vi "IncrementalMove.vi"() -> ()   [LabVIEW 2019]
uses:
  <vilib>/userDefined/High Color/IMAQdx.ctl
  <vilib>/vision/driver/NI_Vision_Acquisition_Software.lvlib
  <vilib>/vision/NI_Vision_Development_Module.lvlib
panel:
  in  "ShowCam":bool
  in  "milliseconds to wait":u32=500
  in  "BadImage":bool
  out "Position_XYZ":string
  out "Gcode":string
  in  "Relative":bool=TRUE
  in  "Z":dbl
  in  "Y":dbl
  in  "X":dbl
  in  "Axis":enum16{"X", "Y", "Z"}(ring)
  out "Image":T1(plugin-control)
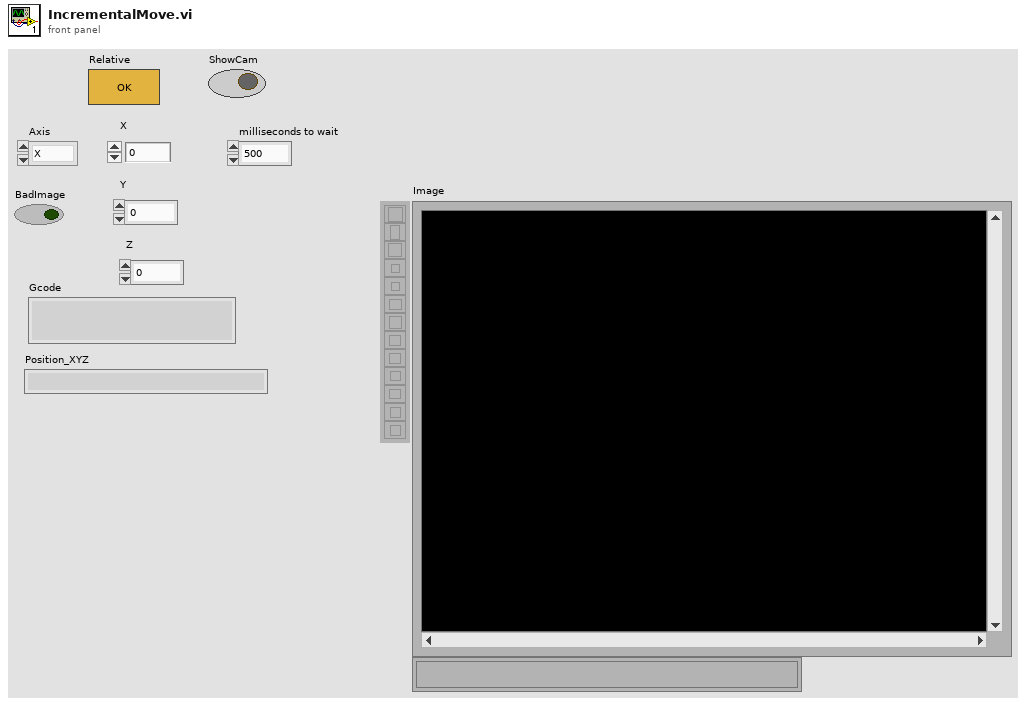
[diagram p1: front panel]
types:
  T1 = typedef "IMAQ Image.ctl" = refnum<image>
  T2 = typedef "IMAQ Circle" = cluster{"Center X":i32, "Center Y":i32, "Inner Radius":i32, "Outer Radius":i32, "Start Angle":dbl, "End Angle":dbl}
  T3 = typedef "IMAQdx.ctl" = refnum<k21>
  T4 = typedef "Image Type" = u32
  T5 = typedef "ROI Descriptor" = cluster{"Global Rectangle":i32[], "Contours":cluster{"ID":enum32{"External", "Internal"}, "Type":u32, "Coordinates":i32[]}[]}
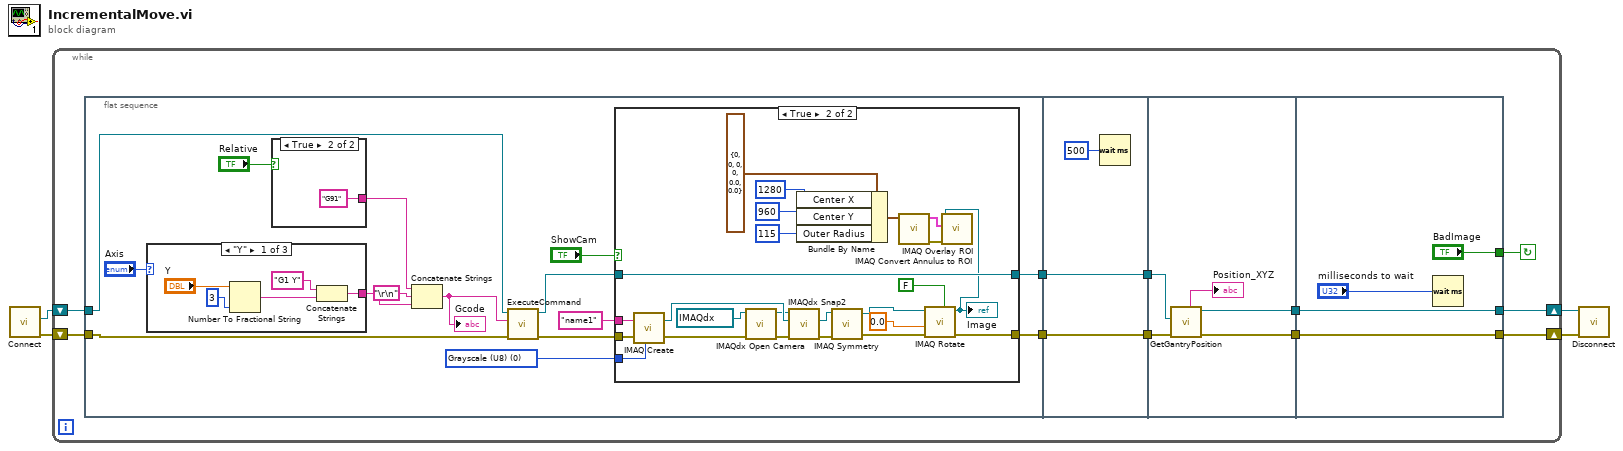
[diagram p0: block diagram]
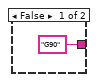
[diagram p3: hidden frame]
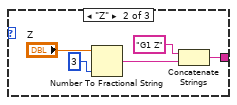
[diagram p4: hidden frame]
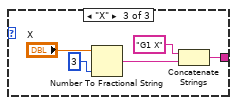
[diagram p5: hidden frame]
diagram:
  n1 = call "Connect.vi"() -> ("error out"=w4:errorcluster, "controller"=w3:refnum<k24>)  [unwired: 10 in]
  n2 = while {
    shift-right: [w13] -> w2
    shift-left: w4 -> [w15]
    shift-right: [w12] -> w1
    shift-left: w3 -> [w14]
    stop <- w11 continue-if-true
    n3 = flat-sequence {
      tunnel: w15 -> [w22]
      tunnel: w14 -> [w21]
      tunnel: [w17] -> w7
      tunnel: [w16] -> w5
      tunnel: [w76] -> w8
      tunnel: w7 -> [w76]
      tunnel: [w75] -> w6
      tunnel: w5 -> [w75]
      tunnel: [w78] -> w10
      tunnel: [w77] -> w9
      tunnel: w8 -> [w80]
      tunnel: w6 -> [w79]
      tunnel: [w84] -> w12
      tunnel: [w85] -> w13
      tunnel: w10 -> [w85]
      tunnel: w9 -> [w84]
      tunnel: ["BadImage"] -> w11
      frame #0 {
        w29 = T4 0 items=["Grayscale (U8)", "Grayscale (I16)", "Grayscale (SGL)", "Complex (CSG)", "RGB (U32)", "HSL (U32)", "RGB (U64)", "Grayscale (U16)"] ("Image Type")
        n4 = case shown="\"Y\"" "Axis" {
          tunnel: [w59 w64 w69] -> w25
          frame "Y" {
            n5 = Number To Fractional String(number="Y", precision (6)=3) -> (F-format string=w63:string)  [unwired: 2 in]
            n6 = Concatenate Strings("G1 Y", w63) -> (w59:string)
          }
          frame "Z" {
            n7 = Number To Fractional String(number="Z", precision (6)=3) -> (F-format string=w68:string)  [unwired: 2 in]
            n8 = Concatenate Strings("G1 Z", w68) -> (w64:string)
          }
          frame "X" {
            n9 = Number To Fractional String(number="X", precision (6)=3) -> (F-format string=w70:string)  [unwired: 2 in]
            n10 = Concatenate Strings("G1 X", w70) -> (w69:string)
          }
        }
        n11 = case shown="True" "Relative" {
          tunnel: ["G90" "G91"] -> w26
          frame False {
          }
          frame True {
          }
        }
        n12 = Concatenate Strings(w26, "\r\n", w25) -> (w23:string)
        "Gcode" <- w23
        n13 = call "ExecuteCommand.vi"("error in (no error)"=w22, "Command Code"=w23, "controller in"=w21) -> ("error out"=w20:errorcluster, "controller out"=w18:refnum<k24>)  [unwired: 6 in, 1 out]
        n14 = case shown="True" "ShowCam" {
          tunnel: "name1" ("Image Name") -> [_ w55]
          tunnel: w29 -> [_ w50]
          tunnel: w20 -> [w32 w47]
          tunnel: [w32 w46] -> w17
          tunnel: [w31 w45] -> w16
          tunnel: w18 -> [w31 w45]
          frame False {
          }
          frame True {
            n15 = call "IMAQ Create"("Image Name"=w55, "Image Type"=w50, "error in (no error)"=w47) -> ("New Image"=w53:T1, "error out"=w51:errorcluster)  [unwired: 2 in]
            n16 = call <vilib>:"IMAQdx Open Camera.vi"("error in"=w51, "Session In"=T3 "cam1") -> ("error out"=w54:errorcluster, "Session Out"=w52:T3)  [unwired: 8 in]
            n17 = call <vilib>:"IMAQdx Snap2.vi"("error in"=w54, "Image In"=w53, "Session In"=w52) -> ("error out"=w44:errorcluster, "Image Out"=w41:T1)  [unwired: 6 in, 1 out]
            n18 = Bundle By Name(cluster=T2 {"Center X"=0, "Center Y"=0, "Inner Radius"=0, "Outer Radius"=0, "Start Angle"=0.0, "End Angle"=0.0} ("Annulus"), "Center X"=1280, "Center Y"=960, "Outer Radius"=115) -> (w40:T2)
            n19 = call "IMAQ Symmetry"("error in (no error)"=w44, "Image Src"=w41) -> ("error out"=w43:errorcluster, "Image Dst Out"=w42:T1)  [unwired: 3 in]
            n20 = call "IMAQ Convert Annulus to ROI"("Annulus"=w40) -> ("error out"=w39:errorcluster, "ROI Descriptor"=w38:T5)  [unwired: 8 in]
            n21 = call "IMAQ Rotate"("Maintain Size"=FALSE, "error in (no error)"=w43, "Angle (degrees)"=sgl 0.0, "Image Src"=w42) -> ("error out"=w46:errorcluster, "Image Dst Out"=w33:T1)  [unwired: 6 in]
            "Image" <- w33
            n22 = call "IMAQ Overlay ROI"("error in (no error)"=w39, "ROI Descriptor"=w38, "Image"=w33) -> ()  [unwired: 7 in, 2 out]
          }
        }
      }
      frame #1 {
        n23 = Wait (ms)(milliseconds to wait=u32 500 ("millisecond timer value")) -> ()  [unwired: 1 out]
      }
      frame #2 {
        n24 = call "GetGantryPosition.vi"("error in (no error)"=w80, "Controller In"=w79) -> ("error out"=w78:errorcluster, "controller out"=w77:refnum<k24>, "Position_XYZ"=→"Position_XYZ":string)  [unwired: 3 in, 4 out]
      }
      frame #3 {
        n25 = Wait (ms)(milliseconds to wait="milliseconds to wait") -> ()  [unwired: 1 out]
      }
    }
  }
  n26 = call "Disconnect.vi"("error in (no error)"=w2, "controller"=w1) -> ()  [unwired: 9 in, 1 out]
